vi "crc_check.vi"(3 "input bit":i16[](array[numeric])) -> (0 "T or F":bool[](array[boolean]), 1 "splited":i16[](array[numeric]))   [LabVIEW 2014]
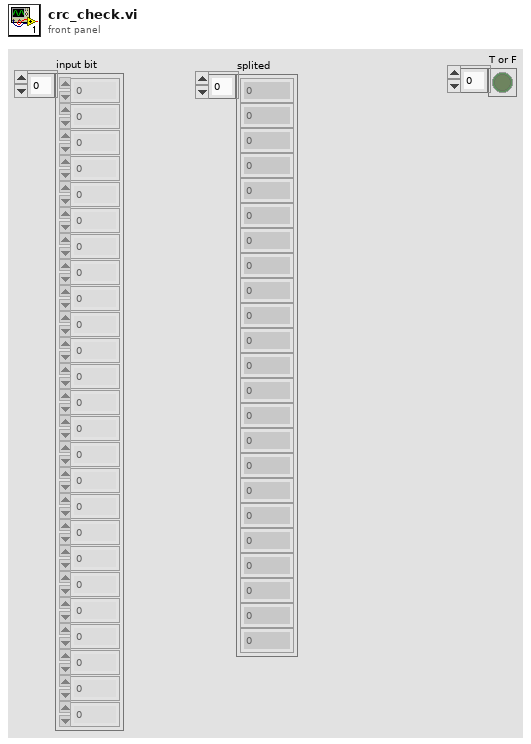
[diagram p1: front panel]
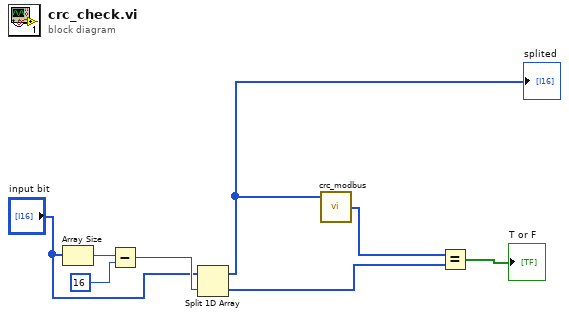
[diagram p0: block diagram]
diagram:
  n1 = Array Size(array="input bit") -> (size(s)=w8:i32)
  n2 = Subtract(x=w8, y=16 ("index")) -> (x-y=w5:i32)
  n3 = Split 1D Array(array="input bit", index=w5) -> (first subarray=w3:i16[], second subarray=w2:i16[])
  "splited" <- w3
  n4 = call "crc_modbus.vi"("input bit"=w3) -> ("crc"=w6:i16[])  [unwired: 3 in, 1 out]
  n5 = Equal?(x=w6, y=w2) -> (x = y?=→"T or F":bool[])
